vi "PXI-4132 Channel Section Page.vi"(8 "error in (no error)":errorcluster, 11 "Node Ptr":T3 format="%.0x") -> (0 "error out":errorcluster)   [LabVIEW 2013, in "PXI-4132 Custom Device.lvlib"]
uses:
  PXI-4132 Custom Device.lvlib
  <vilib>/NI Veristand/Custom Device API/Custom Device Item Ref.ctl
  Channel Sense.ctl
  Channel Type.ctl
  PXI-4132 Global Variable.vi
  <vilib>/NI Veristand/Custom Device API/Get Item Property (I32).vi
  <vilib>/NI Veristand/Custom Device API/Set Item Property (I32).vi
  <vilib>/NI VeriStand/Custom Device API/Custom Device API.lvlib
panel:
  in  "Apply Change":bool
  in  "Channel Type":T1 caption="Channel 0 Sense" items=["Voltage Controlled", "Current Controlled"]
  in  "Channel Sense":T2=1008 caption="Channel 0 Sense" items=["Local"=1008, "Remote"=1009]
  in  "Header":cluster{"Section Name":string}={"Section Name"="Channel Settings"}
  in  "Description":string
  in  "Name":string
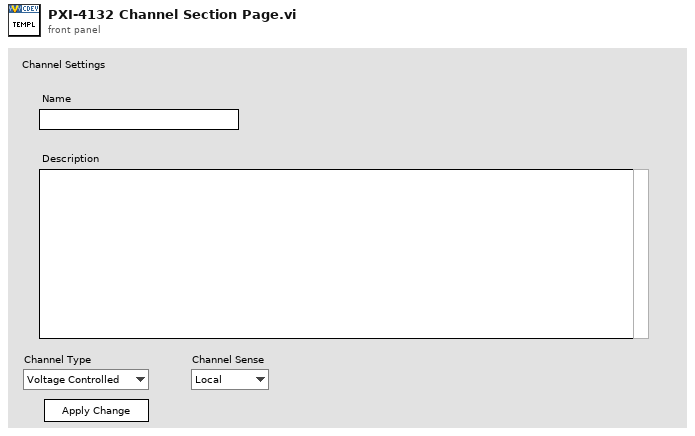
[diagram p1: front panel]
types:
  T1 = typedef "PXI-4132 Custom Device.lvlib/Channel Type.ctl" = i32
  T2 = typedef "PXI-4132 Custom Device.lvlib/Channel Sense.ctl" = i32
  T3 = typedef "Custom Device API.lvlib/Custom Device Item Ref.ctl" = u64
  T4 = enum8{"Enabled", "Disabled", "Disabled and Grayed Out"}
  T5 = typedef "Custom Device API.lvlib/Custom Device Item Info.ctl" = cluster{"Name":string, "Is Channel":bool, "GUID":string, "Is Waveform":bool}
  T6 = typedef "Custom Device API.lvlib/Custom Device Commands.ctl" = enum16{"Default", "Item renamed", "Shutdown", "Dynamic button pressed"}
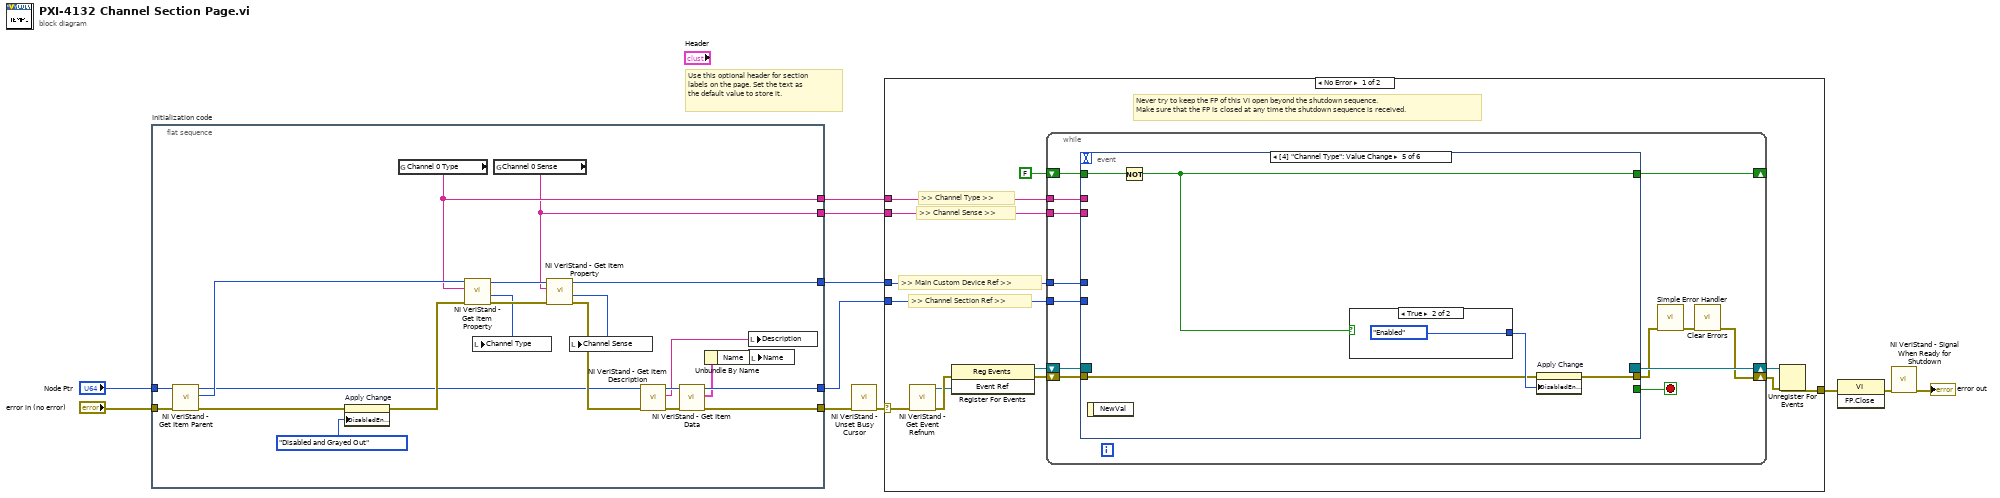
[diagram p0: block diagram]
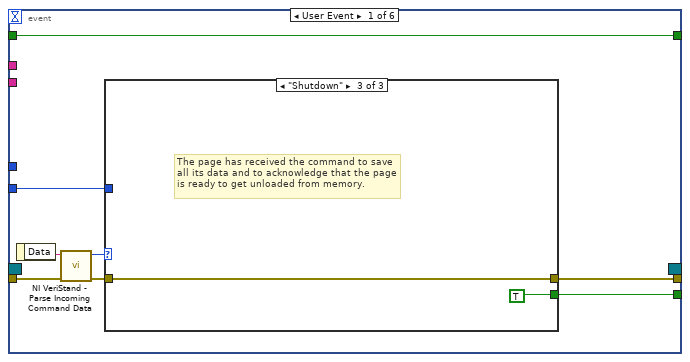
[diagram p2: hidden frame]
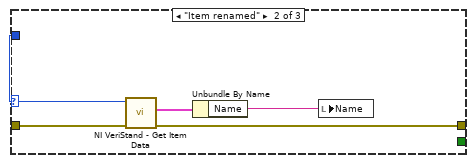
[diagram p4: hidden frame]
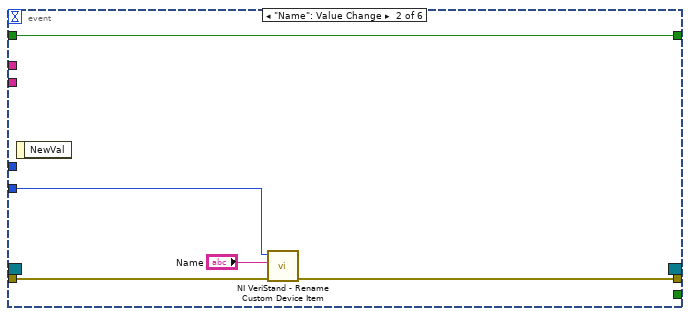
[diagram p5: hidden frame]
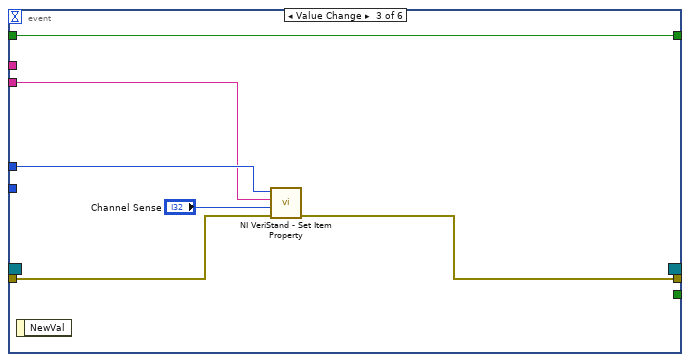
[diagram p6: hidden frame]
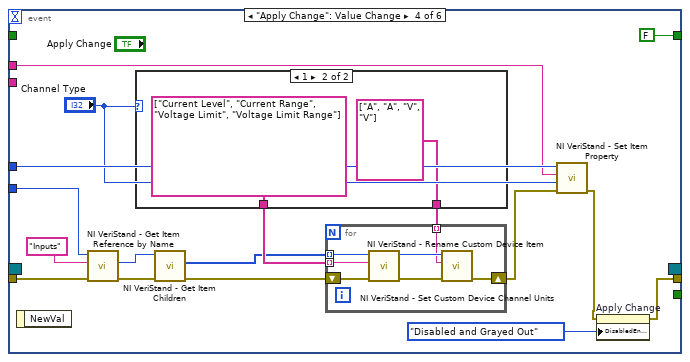
[diagram p7: hidden frame]
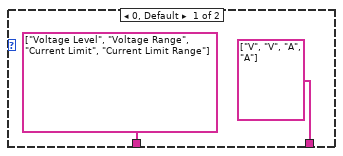
[diagram p8: hidden frame]
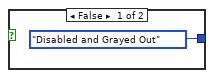
[diagram p9: hidden frame]
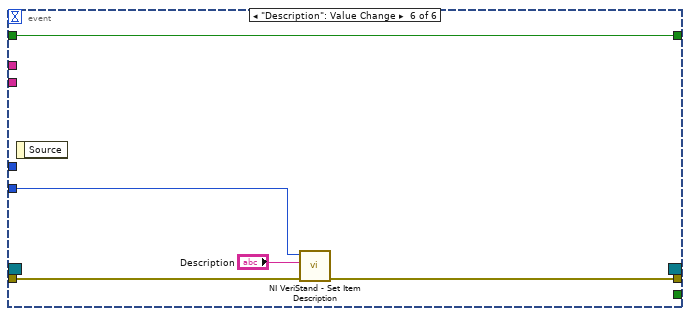
[diagram p10: hidden frame]
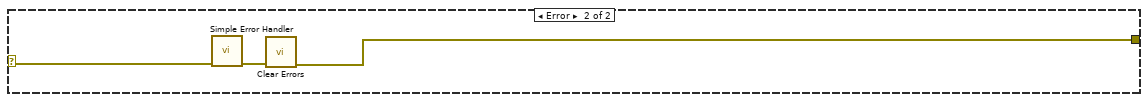
[diagram p11: hidden frame]
diagram:
  # "Use this optional header for section labels on the page. Set the text as the default value to store it."
  n1 = flat-sequence "Initialization code" {
    tunnel: "error in (no error)" -> [w25]
    tunnel: "Node Ptr" -> [w26]
    tunnel: [w27] -> w7
    tunnel: [w33] -> w4
    tunnel: [w17] -> w3
    tunnel: [w13] -> w2
    tunnel: [w14] -> w1
    frame #0 {
      n2 = call <vilib>:"NI VeriStand - Get Item Parent.vi"("error in (no error)"=w25, "Item Ref in"=w26) -> ("error out"=w24:errorcluster, "Parent Ref"=w18:T3, "Item Ref out"=w12:T3)  [unwired: 6 in, 1 out]
      n3 = property on="Apply Change" class="Bool"(error in=w24, "DisabledEnum"=T4."Disabled and Grayed Out" ("Disabled")) -> (error out=w15:errorcluster)  [unwired: 1 in, 1 out]
      n4 = global read "PXI-4132 Global Variable.vi" "Channel 0 Type"() -> (w14:string)
      n5 = call-poly <vilib>:"NI VeriStand - Get Item Property.vi"("error in (no error)"=w15, "Property Name"=w14, "Item Ref in"=w18) -> ("error out"=w22:errorcluster, "Value"=w20:i32, "Item Ref out"=w23:T3)  [unwired: 5 in, 1 out]
      n6 = local write "Channel Type"(w20) -> ()
      n7 = global read "PXI-4132 Global Variable.vi" "Channel 0 Sense"() -> (w13:string)
      n8 = call-poly <vilib>:"NI VeriStand - Get Item Property.vi"("error in (no error)"=w22, "Property Name"=w13, "Item Ref in"=w23) -> ("error out"=w21:errorcluster, "Value"=w19:i32, "Item Ref out"=w17:T3)  [unwired: 5 in, 1 out]
      n9 = local write "Channel Sense"(w19) -> ()
      n10 = call <vilib>:"NI VeriStand - Get Item Description.vi"("error in (no error)"=w21, "Item Ref in"=w12) -> ("error out"=w30:errorcluster, "Description"=w31:string, "Item Ref out"=w32:T3)  [unwired: 7 out]
      n11 = call <vilib>:"NI VeriStand - Get Item Data.vi"("error in (no error)"=w30, "Item Ref in"=w32) -> ("error out"=w27:errorcluster, "Item Info"=w29:T5, "Item Ref out"=w33:T3)  [unwired: 7 out]
      n12 = Unbundle By Name(w29) -> ("Name"=w28:string)
      n13 = local write "Description"(w31) -> ()
      n14 = local write "Name"(w28) -> ()
    }
  }
  n15 = call <vilib>:"NI VeriStand - Unset Busy Cursor.vi"("error in (no error)"=w7) -> ("error out"=w6:errorcluster)  [unwired: 10 out]
  n16 = case shown="No Error" w6 {
    selector: w6 -> [w38 w129]
    tunnel: [w43 w127] -> w11
    tunnel: w4 -> [w39 _]
    tunnel: w3 -> [w37 _]
    tunnel: w2 -> [w36 _]
    tunnel: w1 -> [w35 _]
    frame No Error {
      # ">> Channel Type >>"
      # ">> Channel Sense >>"
      # ">> Main Custom Device Ref >>"
      # ">> Channel Section Ref >>"
      # "Never try to keep the FP of this VI open beyond the shutdown sequence.\nMake sure that the FP is closed at any time the shutdown sequence is received."
      n17 = call <vilib>:"NI VeriStand - Get Event Refnum.vi"("error in (no error)"=w38) -> ("error out"=w46:errorcluster, "Event Ref"=w42:refnum<user-event>)  [unwired: 9 out]
      n18 = register-events(error in=w46, w42) -> (reference out=w40:refnum<event-registration>, error out=w41:errorcluster)  [unwired: 1 in]
      n19 = while {
        tunnel: w39 -> [w55]
        shift-right: [w52] -> w44
        shift-left: w41 -> [w58]
        shift-right: [w59] -> w45
        shift-left: w40 -> [w57]
        tunnel: w37 -> [w51]
        tunnel: w36 -> [w50]
        tunnel: w35 -> [w49]
        shift-right: [w47] -> _
        shift-left: FALSE -> [w48]
        stop <- w56 stop-if-true
        n20 = event shown="[4] \"Channel Type\": Value Change" {
          selector: w57 -> [_ _ _ _ _ _]
          dyn-events: [_ _ _ _ _ _] -> w59
          timeout: _ -> [_ _ _ _ _ _]
          tunnel: w58 -> [w67 w80 w86 w100 w118 w125]
          tunnel: [w63 _ _ _ _ _] -> w56
          tunnel: [w62 w79 w85 w88 w117 w124] -> w54
          tunnel: w55 -> [w61 w78 _ w103 _ w126]
          tunnel: w51 -> [_ _ w83 w94 _ _]
          tunnel: w50 -> [_ _ w82 _ _ _]
          tunnel: w49 -> [_ _ _ w93 _ _]
          tunnel: w48 -> [w60 w76 w81 _ w116 w122]
          tunnel: [w60 w76 w81 FALSE w115 w122] -> w47
          event User Event {
            n21 = event-data() -> ("Data"=w66:string)  [unwired: 1 out]
            n22 = call <vilib>:"NI VeriStand - Parse Incoming Command Data.vi"("error in (no error)"=w67, "Incoming data"=w66) -> ("error out"=w65:errorcluster, "Action"=w64:T6)  [unwired: 8 out]
            n23 = case shown="\"Shutdown\"" w64 {
              tunnel: w65 -> [w68 w73 w74]
              tunnel: [_ _ TRUE] -> w63
              tunnel: [w68 w70 w74] -> w62
              tunnel: w61 -> [_ w72 _]
              frame "Default", Default {
              }
              frame "Item renamed" {
                n24 = call <vilib>:"NI VeriStand - Get Item Data.vi"("error in (no error)"=w73, "Item Ref in"=w72) -> ("error out"=w70:errorcluster, "Item Info"=w71:T5)  [unwired: 8 out]
                n25 = Unbundle By Name(w71) -> ("Name"=w69:string)
                n26 = local write "Name"(w69) -> ()
              }
              frame "Shutdown" {
                # "The page has received the command to save all its data and to acknowledge that the page is ready to get unloaded from memory."
              }
            }
          }
          event "Name": Value Change {
            n27 = event-data() -> ()  [unwired: 2 out]
            n28 = call <vilib>:"NI VeriStand - Rename Custom Device Item.vi"("error in (no error)"=w80, "New Name"="Name", "Item Ref in"=w78) -> ("error out"=w79:errorcluster)  [unwired: 1 in, 7 out]
          }
          event Value Change {
            n29 = event-data() -> ()  [unwired: 2 out]
            n30 = call-poly <vilib>:"NI VeriStand - Set Item Property.vi"("error in (no error)"=w86, "Value"="Channel Sense", "Property Name"=w82, "Item Ref in"=w83) -> ("error out"=w85:errorcluster)  [unwired: 5 in, 2 out]
          }
          event "Apply Change": Value Change {
            n31 = event-data() -> ()  [unwired: 2 out]
            n32 = call <vilib>:"NI VeriStand - Get Item Reference by Name.vi"("error in (no error)"=w100, "Item Name"="Inputs", "Parent Ref in"=w103) -> ("error out"=w101:errorcluster, "Item Ref"=w97:T3)  [unwired: 5 in, 2 out]
            n33 = case shown="1" "Channel Type" {
              tunnel: [string[] ["Voltage Level", "Voltage Range", "Current Limit", "Current Limit Range"] string[] ["Current Level", "Current Range", "Voltage Limit", "Voltage Limit Range"]] -> w99
              tunnel: [string[] ["V", "V", "A", "A"] string[] ["A", "A", "V", "V"]] -> w91
              frame 0, Default {
              }
              frame 1 {
              }
            }
            n34 = call <vilib>:"NI VeriStand - Get Item Children.vi"("error in (no error)"=w101, "Item Ref in"=w97) -> ("error out"=w98:errorcluster, "Child Refs"=w96:T3[])  [unwired: 6 in, 2 out]
            n35 = for {
              tunnel: w99 -> [w110] mode=indexing
              tunnel: w96 -> [w109] mode=indexing
              shift-right: [w106] -> w95
              shift-left: w98 -> [w108]
              tunnel: w91 -> [w104] mode=indexing
              n36 = call <vilib>:"NI VeriStand - Rename Custom Device Item.vi"("error in (no error)"=w108, "New Name"=w110, "Item Ref in"=w109) -> ("error out"=w107:errorcluster, "Item Ref out"=w105:T3)  [unwired: 6 in, 1 out]
              n37 = call <vilib>:"NI VeriStand - Set Custom Device Channel Units.vi"("error in (no error)"=w107, "Units"=w104, "Channel Ref in"=w105) -> ("error out"=w106:errorcluster)  [unwired: 7 in, 1 out]
            }
            n38 = call-poly <vilib>:"NI VeriStand - Set Item Property.vi"("error in (no error)"=w95, "Value"="Channel Type", "Property Name"=w93, "Item Ref in"=w94) -> ("error out"=w89:errorcluster)  [unwired: 5 in, 2 out]
            n39 = property on="Apply Change" class="Bool"(error in=w89, "DisabledEnum"=T4."Disabled and Grayed Out" ("Disabled")) -> (error out=w88:errorcluster)  [unwired: 1 in, 1 out]
          }
          event Value Change {
            n40 = event-data() -> ()  [unwired: 2 out]
            n41 = Not(x=w116) -> (.not. x?=w115:bool)
            n42 = case shown="True" w115 {
              tunnel: [T4."Disabled and Grayed Out" ("Disabled") T4."Enabled" ("Disabled")] -> w119
              frame False {
              }
              frame True {
              }
            }
            n43 = property on="Apply Change" class="Bool"(error in=w118, "DisabledEnum"=w119) -> (error out=w117:errorcluster)  [unwired: 1 in, 1 out]
          }
          event "Description": Value Change {
            n44 = event-data() -> ()  [unwired: 2 out]
            n45 = call <vilib>:"NI VeriStand - Set Item Description.vi"("error in (no error)"=w125, "Description"="Description", "Item Ref in"=w126) -> ("error out"=w124:errorcluster)  [unwired: 8 out]
          }
        }
        n46 = call <vilib>:"Simple Error Handler.vi"("error in (no error)"=w54) -> ("error out"=w53:errorcluster)  [unwired: 1 in, 7 out]
        n47 = call <vilib>:"Clear Errors.vi"("error in (no error)"=w53) -> ("error out"=w52:errorcluster)  [unwired: 6 out]
      }
      n48 = Unregister For Events(event registration refnum=w45, error in=w44) -> (error out=w43:errorcluster)
    }
    frame Error {
      n49 = call <vilib>:"Simple Error Handler.vi"("error in (no error)"=w129) -> ("error out"=w128:errorcluster)  [unwired: 1 in, 7 out]
      n50 = call <vilib>:"Clear Errors.vi"("error in (no error)"=w128) -> ("error out"=w127:errorcluster)  [unwired: 6 out]
    }
  }
  n51 = invoke class="VI" method="FP.Close"(error in=w11) -> (error out=w10:errorcluster)  [unwired: 2 in, 2 out]
  n52 = call <vilib>:"NI VeriStand - Signal When Ready for Shutdown.vi"("error in (no error)"=w10) -> ("error out"=→"error out":errorcluster)  [unwired: 10 out]
